vi "Killswitch Internal.vi"(7 "Writing? (F)":bool, 9 "Write 2nd Button":T2(ring), 10 "Write 1st Button":T2(ring), 11 "Write Mode":T1(ring)) -> ()   [LabVIEW 2010, in "FTC.lvlib"]
uses:
  FTC.lvlib
  <vilib>/NXT/Dual Mode Library/Sound/Tone.vi
  Remote Interface/Remote Interface.lvlib
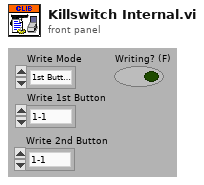
[diagram p1: front panel]
types:
  T1 = enum16{"1st Button Only", "1st AND 2nd Buttons", "1st OR 2nd Button"}
  T2 = enum16{"1-1", "1-2", "1-3", "1-4", "1-5", "1-6", "1-7", "1-8", "1-9", "1-10", "1-11", "1-12", "2-1", "2-2", "2-3", "2-4", "2-5", "2-6", "2-7", "2-8", "2-9", "2-10", "2-11", "2-12", "NXT-L", "NXT-R", "NXT-E", "1-U", "1-UR", "1-R", "1-DR", "1-D", "1-DL", "1-L", "1-UL", "2-U", "2-UR", "2-R", "2-DR", "2-D", "2-DL", "2-L", "2-UL"}
  T3 = typedef "LVHSConnector.ctl" = cluster{"Hardware":string, "Flattened String":string}
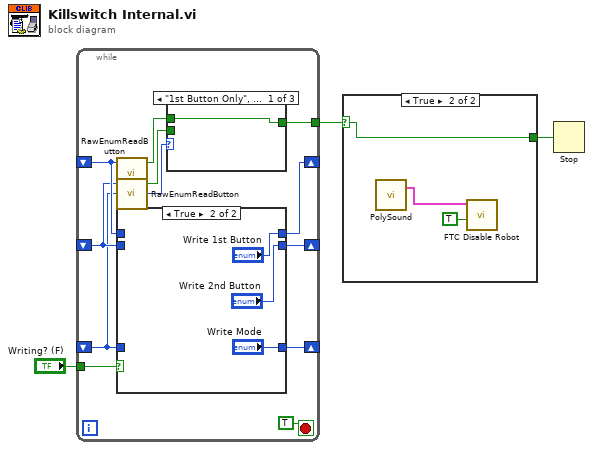
[diagram p0: block diagram]
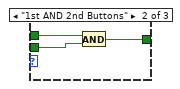
[diagram p3: hidden frame]
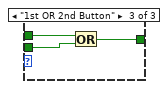
[diagram p4: hidden frame]
diagram:
  n1 = while {
    shift-right: [w11] -> _
    shift-left: _ -> [w8]
    shift-right: [w12] -> _
    shift-left: _ -> [w9]
    tunnel: "Writing? (F)" -> [w13]
    shift-right: [w10] -> _
    shift-left: _ -> [w5]
    tunnel: [w4] -> w2
    stop <- TRUE stop-if-true
    n2 = call "RawEnumReadButton.vi"("Button"=w9) -> ("Pressed?"=w7:bool)  [unwired: 4 in]
    n3 = call "RawEnumReadButton.vi"("Button"=w8) -> ("Pressed?"=w6:bool)  [unwired: 4 in]
    n4 = case shown="True" w13 {
      tunnel: [w24 "Write 1st Button"] -> w12
      tunnel: [w23 "Write 2nd Button"] -> w11
      tunnel: [w22 "Write Mode"] -> w10
      tunnel: w9 -> [w24 _]
      tunnel: w8 -> [w23 _]
      tunnel: w5 -> [w22 _]
      frame False {
      }
      frame True {
      }
    }
    n5 = case shown="\"1st Button Only\", Default" w5 {
      tunnel: w7 -> [w15 w18 w21]
      tunnel: w6 -> [_ w17 w20]
      tunnel: [w15 w16 w19] -> w4
      frame "1st Button Only", Default {
      }
      frame "1st AND 2nd Buttons" {
        n6 = And(x=w18, y=w17) -> (x .and. y?=w16:bool)
      }
      frame "1st OR 2nd Button" {
        n7 = Or(x=w21, y=w20) -> (x .or. y?=w19:bool)
      }
    }
  }
  n8 = case shown="True" w2 {
    selector: w2 -> [_ w30]
    tunnel: [_ w30] -> w1
    frame False {
    }
    frame True {
      n9 = call-poly <vilib>:"PolySound.vi"() -> ("NXT"=w28:T3)  [unwired: 4 in]
      n10 = call <vilib>:"FTC Disable Robot.vi"("Stopped?"=TRUE, "NXT"=w28) -> ()  [unwired: 4 in, 2 out]
    }
  }
  n11 = Stop(stop? (T)=w1) -> ()
